vi "ITestSettings Raw Configuration to Specific Data Type.vi"(8 "error in (no error)":errorcluster, 10 "Raw Configuration Data":refnum<class "String Database.lvclass">[](array[class]), 11 "Band Noise Test Settings in":refnum<class "Band Noise Test Settings.lvclass">=refnum) -> (0 "error out":errorcluster, 3 "Band Noise Test Settings out":refnum<class "Band Noise Test Settings.lvclass">)   [LabVIEW 2016, in "Band Noise Test Settings.lvlib" / "Band Noise Test Settings.lvclass"]
uses:
  Band Noise Test Settings.lvclass
  Controls/Band Noise Settings Cluster.ctl
  Plugins/String Database.lvlibp/String Database.lvclass
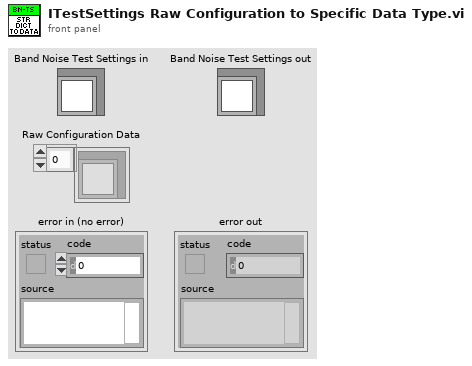
[diagram p1: front panel]
types:
  T1 = typedef "Band Noise Test Settings.lvlib/Band Noise Test Settings.lvclass/Band Noise Settings Cluster.ctl" = cluster{"Frequency":dbl, "Reference Level":dbl, "Span":dbl}
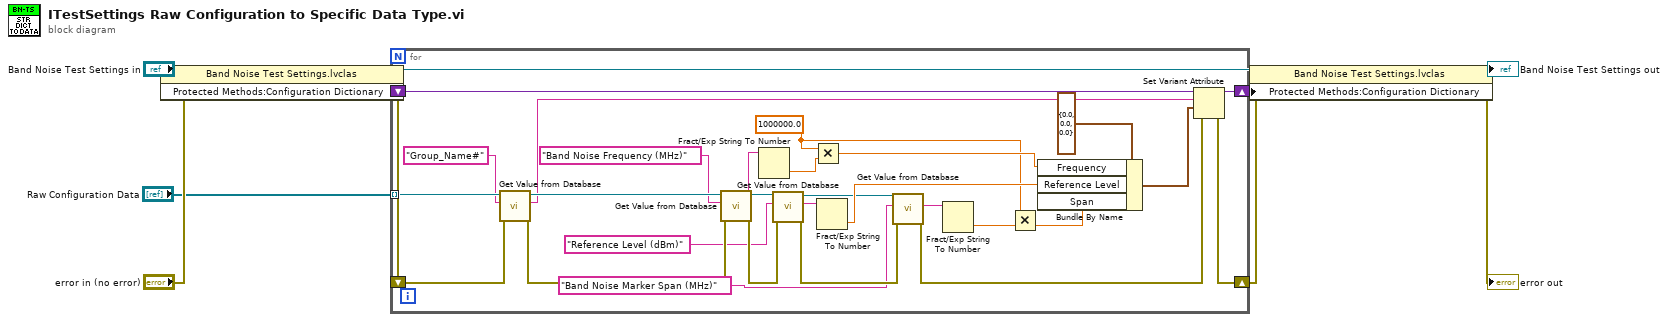
[diagram p0: block diagram]
diagram:
  n1 = property class="Band Noise Test Settings.lvclas"(reference="Band Noise Test Settings in", error in="error in (no error)") -> (reference out=w4:refnum<class "Band Noise Test Settings.lvclass">, error out=w9:errorcluster, "Protected Methods:Configuration Dictionary"=w7)
  n2 = for {
    shift-right: [w37] -> w6
    shift-left: w9 -> [w34]
    shift-right: [w36] -> w2
    shift-left: w7 -> [w38]
    tunnel: "Raw Configuration Data" -> [w35] mode=indexing
    w11 = 1000000.0 ("x")
    n3 = call "Get Value from Database.vi"("error in (no error)"=w34, "Entry Name"="Group_Name#", "Message in"=w35) -> ("error out"=w31:errorcluster, "Entry Value"=w28:string, "Message out"=w32:refnum<class "String Database.lvclass">)  [unwired: 5 in, 1 out]
    n4 = call "Get Value from Database.vi"("error in (no error)"=w31, "Entry Name"="Band Noise Frequency (MHz)", "Message in"=w32) -> ("error out"=w29:errorcluster, "Entry Value"=w25:string, "Message out"=w30:refnum<class "String Database.lvclass">)  [unwired: 5 in, 1 out]
    n5 = Fract/Exp String To Number(string=w25) -> (number=w24:dbl)  [unwired: 3 in, 1 out]
    n6 = call "Get Value from Database.vi"("error in (no error)"=w29, "Entry Name"="Reference Level (dBm)", "Message in"=w30) -> ("error out"=w17:errorcluster, "Entry Value"=w22:string, "Message out"=w18:refnum<class "String Database.lvclass">)  [unwired: 5 in, 1 out]
    n7 = Multiply(x=w11, y=w24) -> (x*y=w23:dbl)
    n8 = Fract/Exp String To Number(string=w22) -> (number=w21:dbl)  [unwired: 3 in, 1 out]
    n9 = call "Get Value from Database.vi"("error in (no error)"=w17, "Entry Name"="Band Noise Marker Span (MHz)", "Message in"=w18) -> ("error out"=w16:errorcluster, "Entry Value"=w14:string)  [unwired: 5 in, 2 out]
    n10 = Fract/Exp String To Number(string=w14) -> (number=w13:dbl)  [unwired: 3 in, 1 out]
    n11 = Multiply(x=w11, y=w13) -> (x*y=w12:dbl)
    n12 = Bundle By Name(cluster=T1 {"Frequency"=0.0, "Reference Level"=0.0, "Span"=0.0} ("Band Noise Test Settings"), "Frequency"=w23, "Reference Level"=w21, "Span"=w12) -> (w27:T1)
    n13 = Set Variant Attribute(Variant=w38, name=w28, value=w27, error in=w16) -> (Variant out=w36:variant, error out=w37:errorcluster)  [unwired: 1 out]
  }
  n14 = property class="Band Noise Test Settings.lvclas"(reference=w4, error in=w6, "Protected Methods:Configuration Dictionary"=w2) -> (reference out=→"Band Noise Test Settings out":refnum<class "Band Noise Test Settings.lvclass">, error out=→"error out":errorcluster)
